vi "Run Service.vi"() -> ()   [LabVIEW 2020, in "MeasurementLink Measurement Server.lvlib"]
uses:
  MeasurementLink Measurement Server.lvlib
  <vilib>/gRPC/LabVIEW gRPC Servicer/Servicer/Servicer.lvclass
  MeasurementLink Measurement Server Internal/MeasurementLink Measurement Server Internal.lvlib
  MeasurementLink Measurement Server Internal/RPC Service/MeasurementService/MeasurementService.lvclass
  <vilib>/MeasurementLink/Discovery Client/MeasurementLink Discovery Client.lvlib
panel:
  out "Listening Port":i32
  in  "Stop":bool
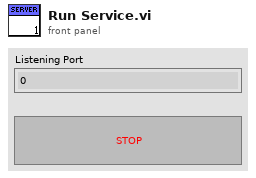
[diagram p1: front panel]
types:
  T1 = enum32{"Invalid", "Standard", "Closed", "Hidden", "Minimized", "Maximized"}
  T2 = typedef "grpc-lvsupport-release.lvlib/grpcId.ctl" = u64
  T3 = typedef "MeasurementLink Discovery Client.lvlib/ni_measurementlink_discovery_v1_RegisterServiceResponse.ctl" = cluster{"registration_id":string}
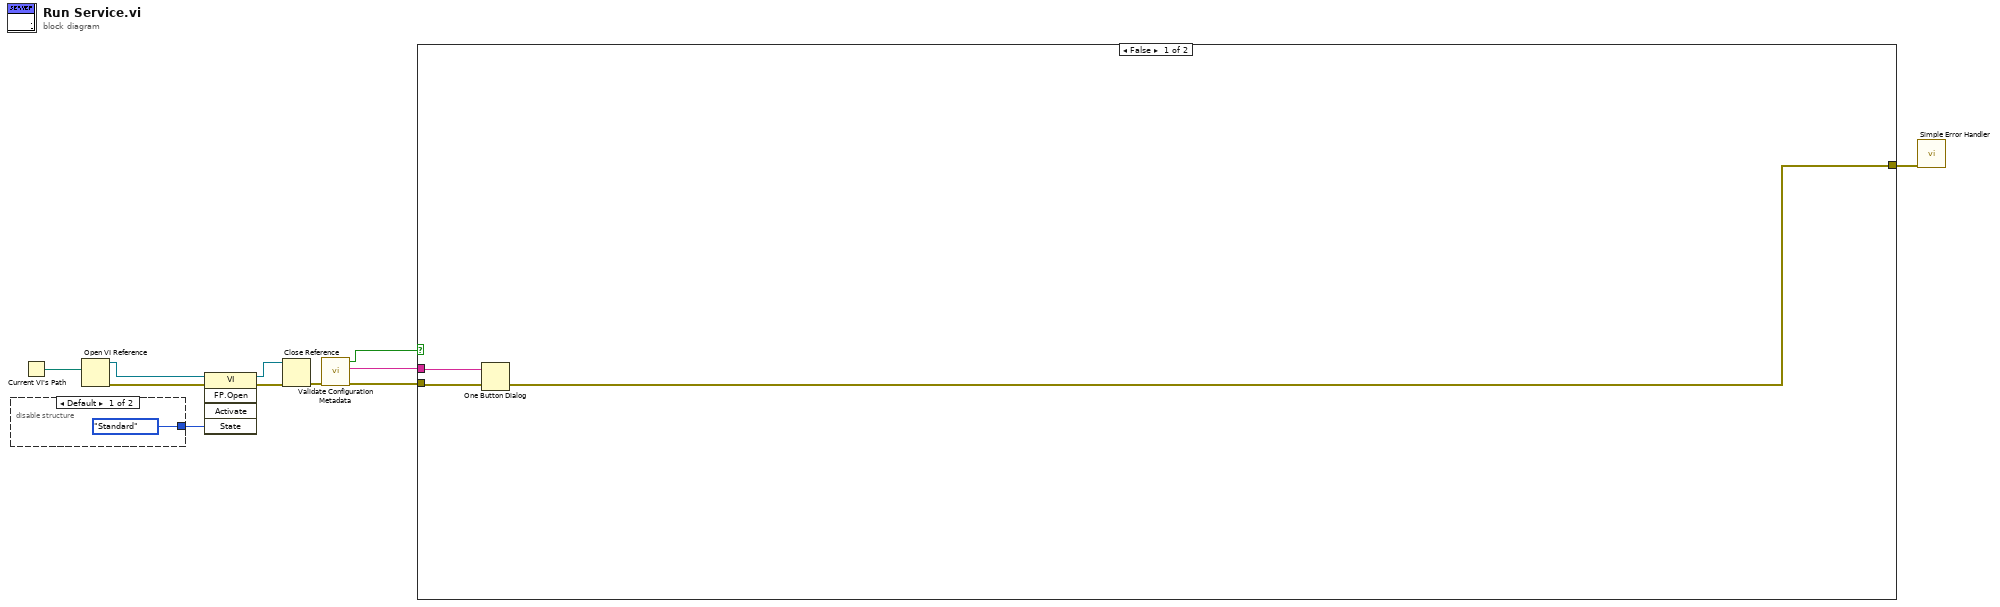
[diagram p0: block diagram]
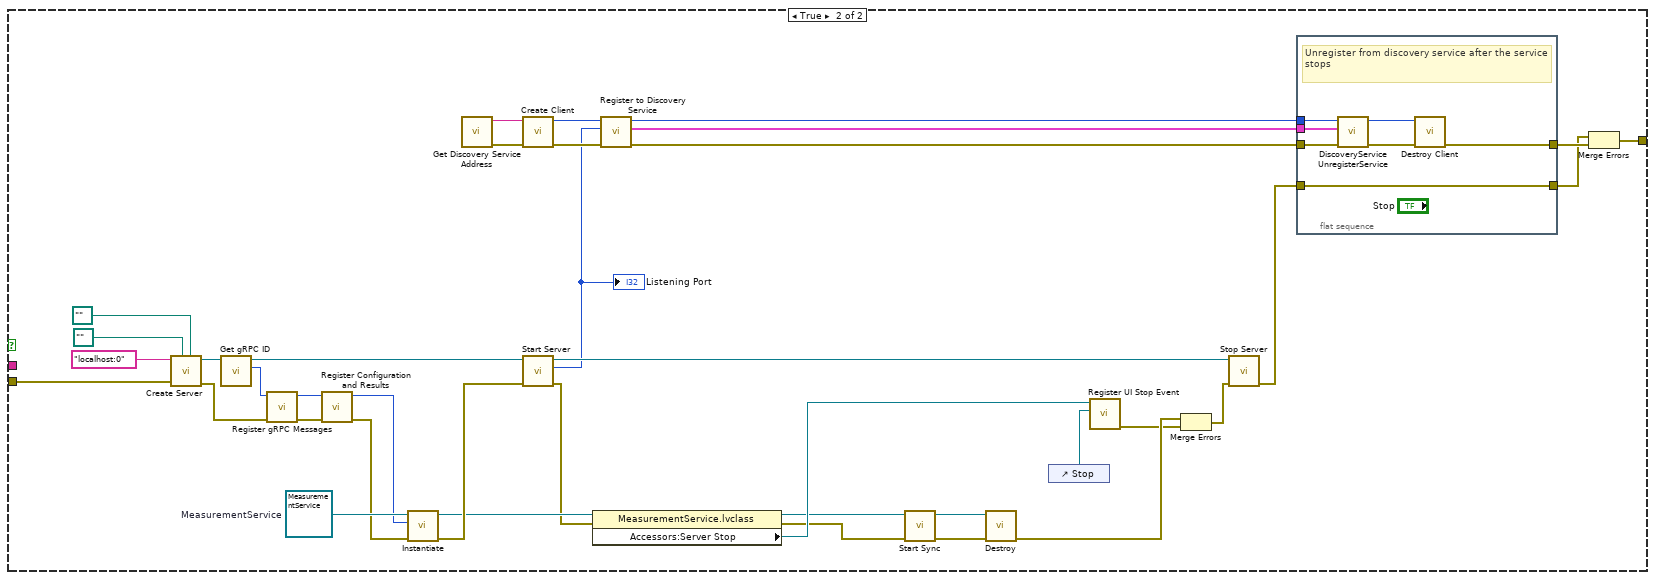
[diagram p2: hidden frame]
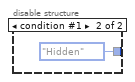
[diagram p3: hidden frame]
diagram:
  n1 = disable-structure shown="Default" {
    disable-tunnel: [T1."Standard" ("State") T1."Hidden" ("State")] -> w6
    frame condition #0 (active) {
    }
    frame condition #1 {
    }
  }
  n2 = Current VI's Path() -> (path=w10:path)
  n3 = Open VI Reference(vi path=w10) -> (vi reference=w7:refnum<vi>, error out=w9:errorcluster)  [unwired: 5 in]
  n4 = invoke class="VI" method="FP.Open"(reference=w7, error in=w9, "State"=w6) -> (reference out=w5:refnum<vi>, error out=w8:errorcluster)  [unwired: 2 in, 3 out]
  n5 = Close Reference(reference=w5, error in (no error)=w8) -> (error out=w4:errorcluster)
  n6 = call "Validate Configuration Metadata.vi"("error in (no error)"=w4) -> ("error out"=w3:errorcluster, "Invalid Parameters"=w1:string, "Is Metadata Valid"=w2:bool)  [unwired: 8 in]
  n7 = case shown="False" w2 {
    tunnel: [w14 w34] -> w11
    tunnel: w3 -> [w14 w16]
    tunnel: w1 -> [w15 _]
    frame False {
      n8 = One Button Dialog(message=w15) -> ()  [unwired: 1 in, 1 out]
    }
    frame True {
      w44 = refnum<class "MeasurementService.lvclass"> refnum  # MeasurementService
      n9 = call <vilib>:"Create Server.vi"("Server Key File (.key)"=path "", "Server Certificate File (.crt)"=path "", "error in"=w16, "Server Address"="localhost:0") -> ("error out"=w47:errorcluster, "gRPC Server out"=w49:refnum<class "Servicer.lvclass">)  [unwired: 6 in]
      n10 = call <vilib>:"Get gRPC ID.vi"("OOP Server in"=w49) -> ("gRPC ID"=w48:T2, "OOP Server out"=w43:refnum<class "Servicer.lvclass">)  [unwired: 9 in]
      n11 = call "Register gRPC Messages.vi"("error in (no error)"=w47, "gRPC ID"=w48) -> ("error out"=w30:errorcluster, "gRPC ID Out"=w31:T2)  [unwired: 8 in]
      n12 = call "Register Configuration and Results.vi"("error in (no error)"=w30, "gRPC ID"=w31) -> ("error out"=w29:errorcluster, "gRPC ID Out"=w27:T2)  [unwired: 8 in]
      n13 = call-dynamic "Instantiate.vi"("error in"=w29, "gRPCid"=w27, "iService"=w44) -> ("error out"=w23:errorcluster, "iService"=w22:refnum<class "MeasurementService.lvclass">)  [unwired: 7 in]
      n14 = call "Get Discovery Service Address.vi"() -> ("error out"=w18:errorcluster, "address"=w17:string)  [unwired: 10 in]
      n15 = call <vilib>:"Create Client.vi"("error in"=w18, "address"=w17) -> ("error out"=w40:errorcluster, "gRPC ID Out"=w41:T2)  [unwired: 8 in]
      n16 = call <vilib>:"Start Server.vi"("error in"=w23, "gRPC Server in"=w43) -> ("error out"=w21:errorcluster, "Listening Port"=w28:i32, "gRPC Server out"=w53:refnum<class "Servicer.lvclass">)  [unwired: 7 in]
      "Listening Port" <- w28
      n17 = property class="MeasurementService.lvclass"(reference=w22, error in=w21) -> (reference out=w19:refnum<class "MeasurementService.lvclass">, error out=w20:errorcluster, "Accessors:Server Stop"=w24:refnum<user-event>)
      n18 = call "Register to Discovery Service.vi"("error in"=w40, "PortNumber"=w28, "gRPC ID"=w41) -> ("error out"=w38:errorcluster, "Response Data"=w37:T3, "gRPC ID out"=w39:T2)  [unwired: 6 in]
      n19 = call-dynamic "Start Sync.vi"("error in"=w20, "gRPC Server in"=w19) -> ("error out"=w46:errorcluster, "gRPC Server out"=w45:refnum<class "MeasurementService.lvclass">)  [unwired: 8 in]
      n20 = call-dynamic "Destroy.vi"("error in (no error)"=w46, "SignalGeneratorService in"=w45) -> ("error out"=w26:errorcluster)  [unwired: 8 in, 1 out]
      n21 = control-ref of="Stop"() -> (w36:refnum<vi>)
      n22 = call "Register UI Stop Event.vi"("Stop Button [ref]"=w36, "Server Stop"=w24) -> ("error out"=w25:errorcluster)  [unwired: 9 in]
      n23 = Merge Errors(w26, w25) -> (w42:errorcluster)
      n24 = call <vilib>:"Stop Server.vi"("error in"=w42, "gRPC Server in"=w53) -> ("error out"=w32:errorcluster)  [unwired: 9 in]
      n25 = flat-sequence {
        tunnel: w39 -> [w60]
        tunnel: w38 -> [w59]
        tunnel: w37 -> [w58]
        tunnel: [w55] -> w35
        tunnel: [w54] -> w33
        tunnel: w32 -> [w54]
        frame #0 {
          # "Unregister from discovery service after the service stops"
          n26 = call <vilib>:"DiscoveryService UnregisterService.vi"("error in"=w59, "Request Data"=w58, "gRPC ID"=w60) -> ("error out"=w56:errorcluster, "gRPC ID out"=w57:T2)  [unwired: 6 in, 1 out]
          n27 = call <vilib>:"Destroy Client.vi"("error in"=w56, "gRPC ID"=w57) -> ("error out"=w55:errorcluster)  [unwired: 9 in]
        }
      }
      n28 = Merge Errors(w33, w35) -> (w34:errorcluster)
    }
  }
  n29 = call <vilib>:"Simple Error Handler.vi"("error in (no error)"=w11) -> ()  [unwired: 4 in, 5 out]
